vi "Set XY Graph To S.D Plot.vi"(8 "Color":u32(colorbox)=37103, 9 "Number":i32, 10 "Plot Start":i32, 11 "XY Graph Reference In":refnum<vi>) -> (3 "XY Graph Reference Out":refnum<vi>)   [LabVIEW 2024]
uses:
  Set XY Graph Line Color.vi
  Set XY Graph Bar Style.vi
  Set XY Graph Interpolation Style.vi
  Set XY Graph Point Style.vi
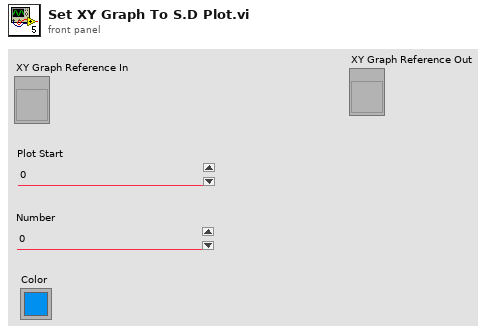
[diagram p1: front panel]
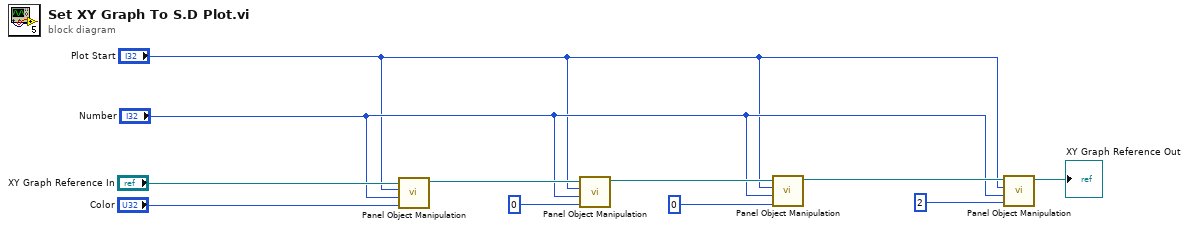
[diagram p0: block diagram]
diagram:
  n1 = call-poly "Panel Object Manipulation.vi"("Color"="Color", "Number"="Number", "Active Plot Start"="Plot Start", "XY Graph Reference In"="XY Graph Reference In") -> ("XY Graph Reference Out"=w9:refnum<vi>)  [unwired: 7 in]
  n2 = call-poly "Panel Object Manipulation.vi"("Bar Style"=u8 0, "Number"="Number", "Active Plot Start"="Plot Start", "XY Graph Reference In"=w9) -> ("XY Graph Reference Out"=w7:refnum<vi>)  [unwired: 7 in]
  n3 = call-poly "Panel Object Manipulation.vi"("InterPolation Style"=u8 0 ("Bar Style"), "Number"="Number", "Active Plot Start"="Plot Start", "XY Graph Reference In"=w7) -> ("XY Graph Reference Out"=w5:refnum<vi>)  [unwired: 7 in]
  n4 = call-poly "Panel Object Manipulation.vi"("Point Style"=u8 2, "Number"="Number", "Active Plot Start"="Plot Start", "XY Graph Reference In"=w5) -> ("XY Graph Reference Out"=→"XY Graph Reference Out":refnum<vi>)  [unwired: 7 in]
